vi "UDP Listener Display Values.vi"() -> ()   [LabVIEW 2014]
doc: "This example simple creates UDP listener on specific and read data from specific host (by IP address). Then from received string convert values into real numbers and showed them in chart."
panel:
  out "Waveform Chart":cluster{dbl, dbl, dbl}(graph)
  out "data out":string
  in  "Stop":bool
  # "Overview: Demonstrates the use of the UDP functions to receive data over a UDP connection.\nInstructions:\n1. Ensure Simple UDP - Sender.vi is already running.\n2. Run the VI.\n3. Click Stop to stop the VI."
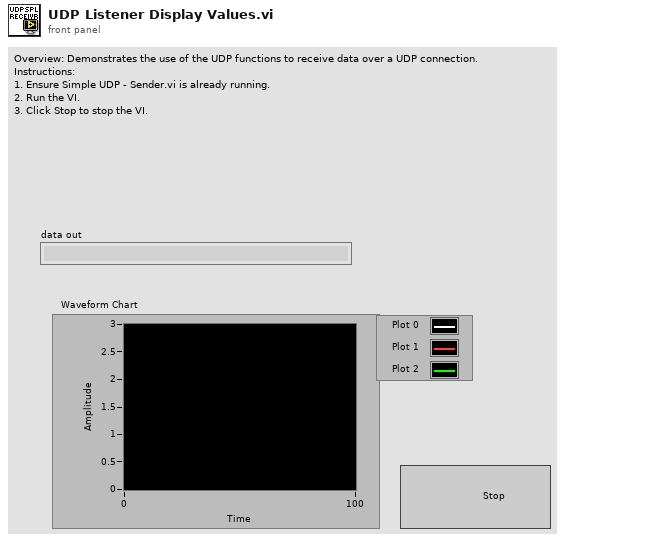
[diagram p1: front panel]
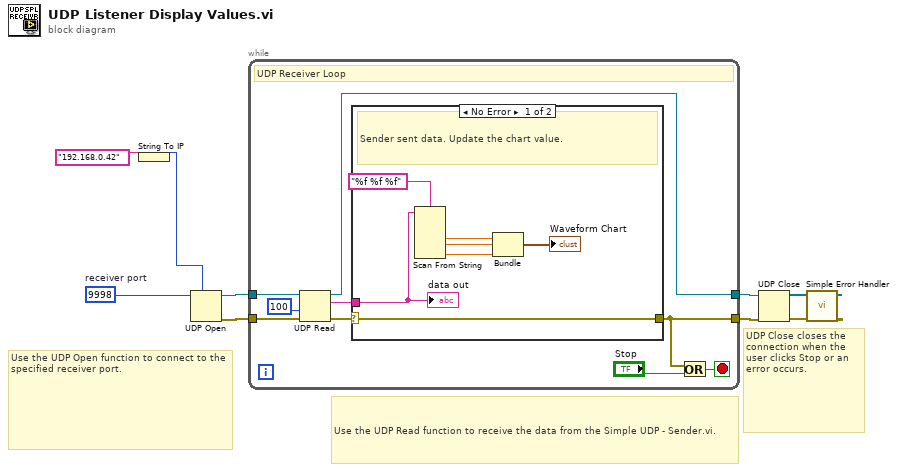
[diagram p0: block diagram]
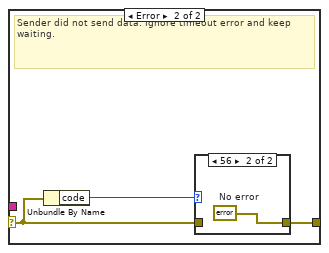
[diagram p2: hidden frame]
diagram:
  w3 = u16 9998  # receiver port
  # "UDP Close closes the connection when the user clicks Stop or an error occurs."
  # "Use the UDP Open function to connect to the specified receiver port."
  # "Use the UDP Read function to receive the data from the Simple UDP - Sender.vi."
  n1 = String To IP(1:"192.168.0.42" ("name")) -> (0:w1:u32)
  n2 = UDP Open(7:w1, 11:w3) -> (port=w4:refnum<k16>, 0:w5:errorcluster)  [unwired: 3 in, 1 out]
  n3 = while {
    tunnel: w4 -> [w17]
    tunnel: [w9] -> w8
    tunnel: w5 -> [w14]
    tunnel: [w10] -> w6
    stop <- w15 stop-if-true
    # "UDP Receiver Loop"
    n4 = UDP Read(connection ID=w17, timeout ms (25000)=100, 8:w14) -> (data out=w12:string, error out=w11:errorcluster, 3:w9:refnum<k16>)  [unwired: 3 out]
    n5 = case shown="No Error" w11 {
      selector: w11 -> [w24 w26]
      tunnel: w12 -> [w22 _]
      tunnel: [w24 w25] -> w10
      frame No Error {
        # "Sender sent data. Update the chart value."
        n6 = Scan From String(format string="%f %f %f", input string=w22) -> (output 1=w21:dbl, output 2=w20:dbl, output 3=w19:dbl)  [unwired: 5 in, 3 out]
        n7 = Bundle(w21, w20, w19) -> (→"Waveform Chart":cluster{dbl, dbl, dbl})  [unwired: 1 in]
        "data out" <- w22
      }
      frame Error {
        # "Sender did not send data. Ignore timeout error and keep waiting."
        n8 = Unbundle By Name(w26) -> ("code"=w27:i32)
        n9 = case shown="56" w27 {
          tunnel: w26 -> [w28 _]
          tunnel: [w28 w29] -> w25
          frame Default {
          }
          frame 56 {
            w29 = errorcluster {"status"=FALSE, "code"=0, "source"=""}  # No error
          }
        }
      }
    }
    n10 = Or(x=w10, y="Stop") -> (x .or. y?=w15:bool)
  }
  n11 = UDP Close(connection ID=w8, 8:w6) -> (error out=w7:errorcluster)  [unwired: 1 out]
  n12 = call <vilib>:"Simple Error Handler.vi"("error in (no error)"=w7) -> ()  [unwired: 1 in, 8 out]
